vi "Write DO.vi"(8 "error in (no error)":errorcluster, 10 "Array":i32[](array[numeric]), 11 "DIO in":refnum<class "DIO.lvclass">) -> (0 "error out":errorcluster, 3 "DIO out":refnum<class "DIO.lvclass">)   [LabVIEW 2015, in "DIO.lvclass"]
uses:
  DIO.lvclass
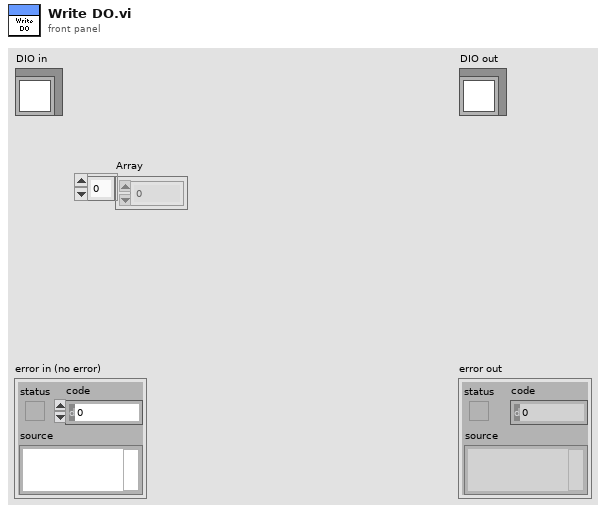
[diagram p1: front panel]
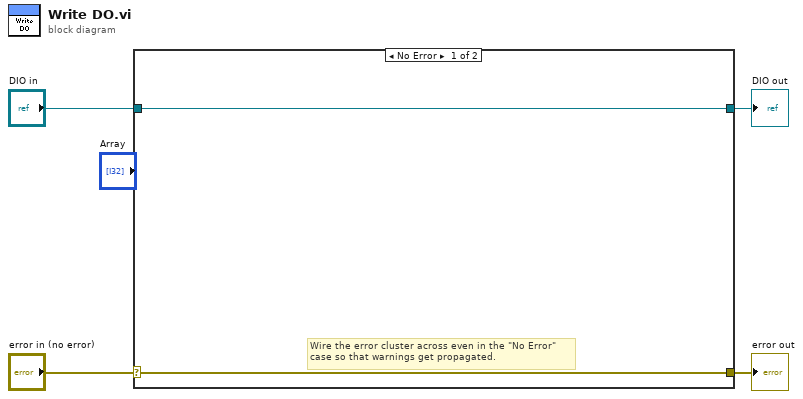
[diagram p0: block diagram]
diagram:
  n1 = case shown="No Error" "error in (no error)" {
    selector: "error in (no error)" -> [w5 w8]
    tunnel: [w5 w8] -> w3
    tunnel: [w6 w7] -> w1
    tunnel: "DIO in" -> [w6 w7]
    frame No Error {
      # "Wire the error cluster across even in the \"No Error\"\ncase so that warnings get propagated."
    }
    frame Error {
    }
  }
  "error out" <- w3
  "DIO out" <- w1
